vi "init_chessboard.vi"(8 "error in (no error)":errorcluster, 10 "starting_square":T1, 11 "chessboard_size":u8) -> (0 "error out":errorcluster, 3 "chessboard (populated)":T2[][](array[typedef]))   [LabVIEW 2020, in "core.lvlib"]
uses:
  core.lvlib
  core_data/core_data.ctl
  core_data/tour_in_progress.ctl
  core_data/chessboard_index.ctl
  core_data/chess_square.ctl
  core_data/neighbour_square.ctl
  core_data/core_data.lvlib
  PTRL/errors/errors.lvlib
panel:
  out "no. of neighbours":i32[][](array[numeric])
  out "no. of rows and columns":i32[](array[numeric])
  out "chessboard (not populated)":T2[][](array[typedef])
  out "chess_square":T2
  out "core_data":T4
  # "Development\ncontrols/indicators useful for development and testing, but which are not outputs of the VI"
  # "Input\nInputs to the VI"
  # "Output\nOutputs of the VI"
  # "Description\n\nBlank VI with error handling case. \n\nSummarize the use of this VI in this space."
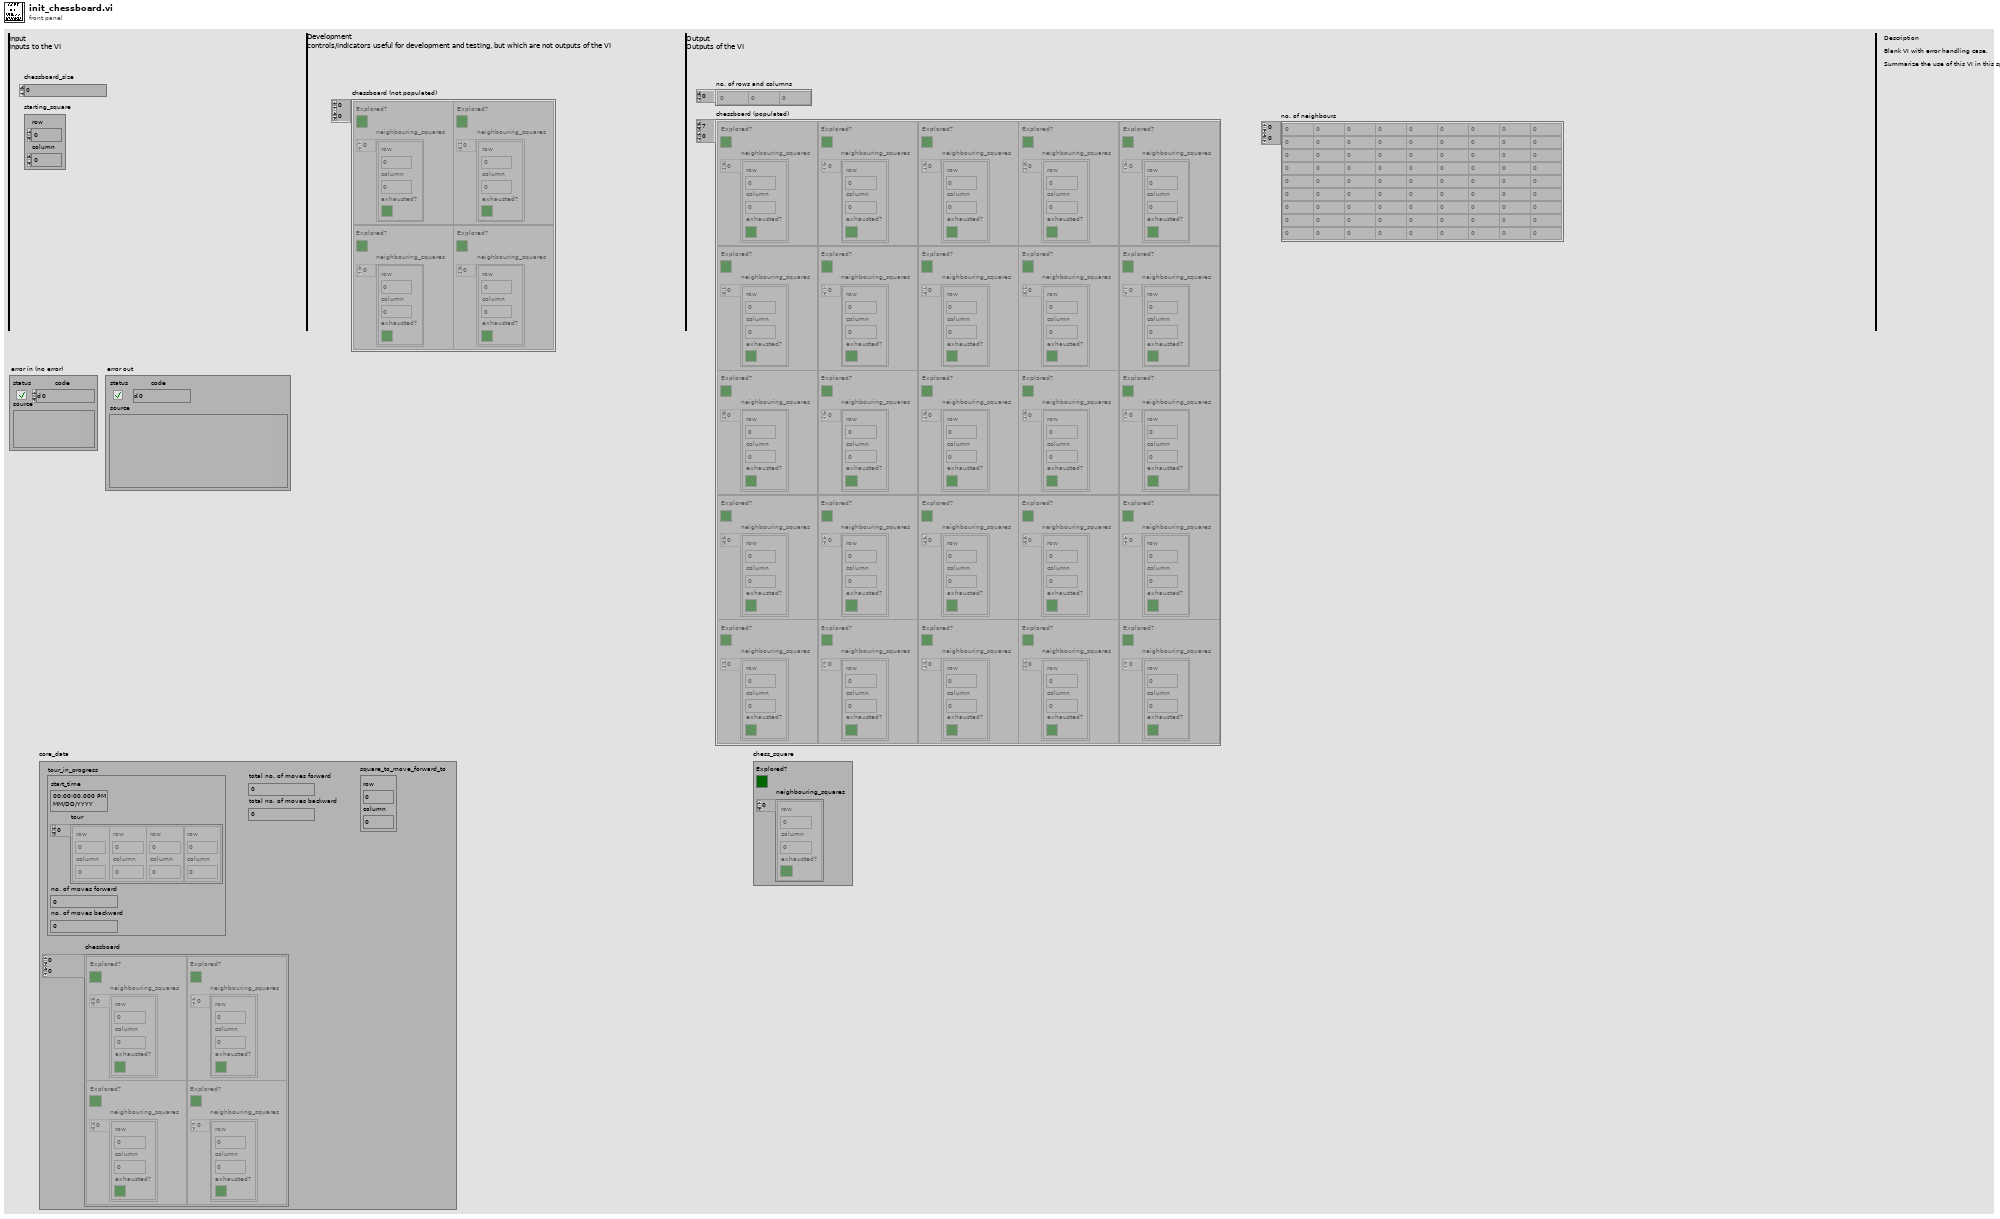
[diagram p1: front panel]
types:
  T1 = typedef "core.lvlib/core_data.lvlib/chessboard_index.ctl" = cluster{"row":u8, "column":u8}
  T2 = typedef "core.lvlib/core_data.lvlib/chess_square.ctl" = cluster{"Explored?":bool, "neighbouring_squares":T3[]}
  T3 = typedef "core.lvlib/core_data.lvlib/neighbour_square.ctl" = cluster{"row":u8, "column":u8, "exhausted?":bool}
  T4 = typedef "core.lvlib/core_data.lvlib/core_data.ctl" = cluster{"tour_in_progress":T5, "total no. of moves forward":u64, "total no. of moves backward":u64, "chessboard":T2[][], "square_to_move_forward_to":T1}
  T5 = typedef "core.lvlib/core_data.lvlib/tour_in_progress.ctl" = cluster{"start_time":timestamp, "tour":T1[], "no. of moves forward":u64, "no. of moves backward":u64}
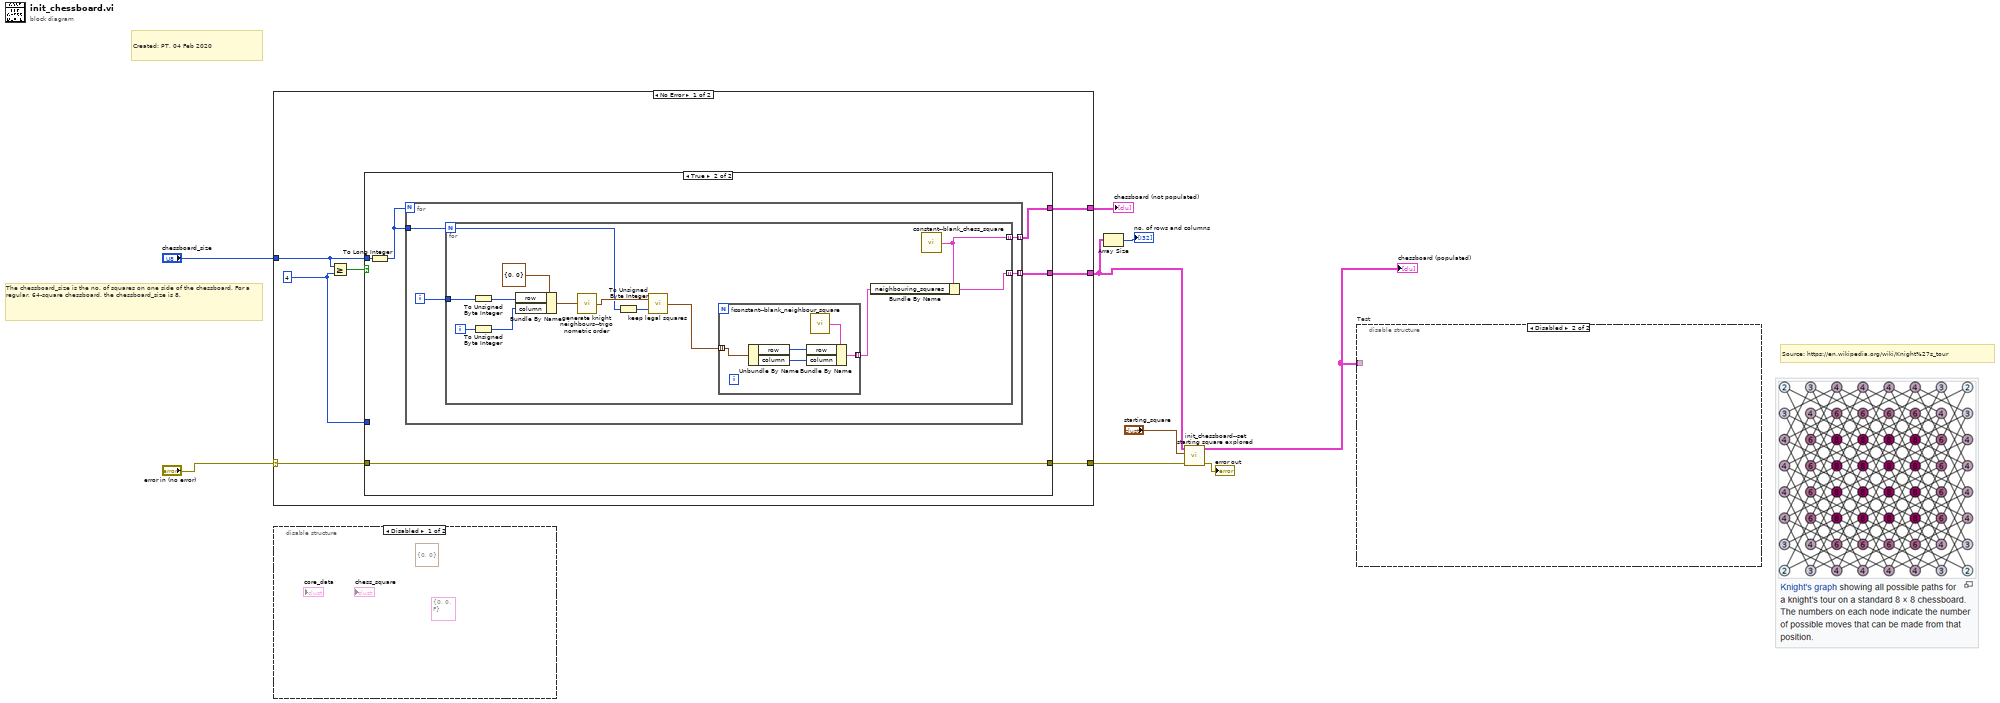
[diagram p0: block diagram]
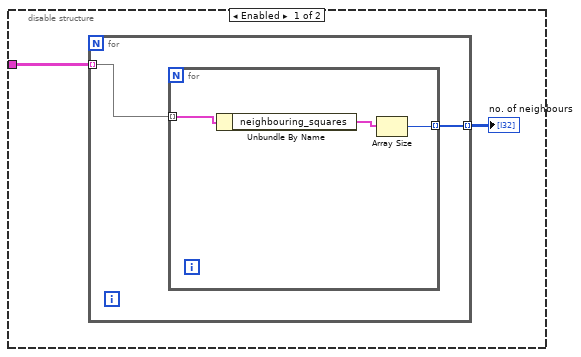
[diagram p2: hidden frame]
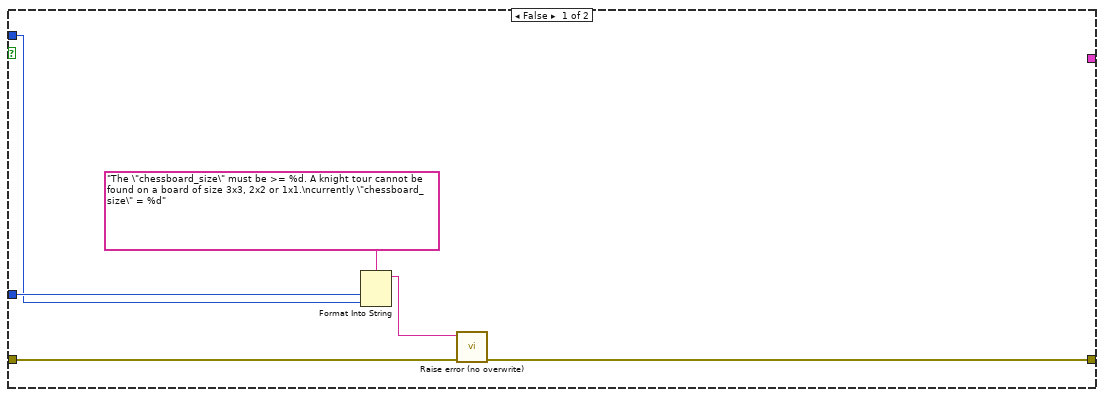
[diagram p4: hidden frame]
diagram:
  # "Source: https://en.wikipedia.org/wiki/Knight%27s_tour"
  # "The chessboard_size is the no. of squares on one side of the chessboard. For a regular, 64-square chessboard, the chessboard_size is 8."
  # "Created: PT, 04 Feb 2020"
  n1 = case shown="No Error" "error in (no error)" {
    selector: "error in (no error)" -> [w14 w50]
    tunnel: [w13 w50] -> w3
    tunnel: "chessboard_size" -> [w16 _]
    tunnel: [w11 _] -> w7
    tunnel: [w10 _] -> w5
    frame No Error {
      w12 = u8 4 ("y")
      n2 = Greater Or Equal?(x=w16, y=w12) -> (x >= y?=w15:bool)
      n3 = case shown="True" w15 {
        tunnel: w16 -> [w17 w27]
        tunnel: w14 -> [w22 w25]
        tunnel: [w21 w25] -> w13
        tunnel: w12 -> [w18 _]
        tunnel: [_ w24] -> w11
        tunnel: [_ w23] -> w10
        frame False {
          n4 = Format Into String(format string="The \"chessboard_size\" must be >= %d. A knight tour cannot be found on a board of size 3x3, 2x2 or 1x1.\ncurrently \"chessboard_size\" = %d", w18, w17) -> (resulting string=w19:string)  [unwired: 2 in, 1 out]
          n5 = call "Raise error (no overwrite).vi"("error in"=w22, "error message (\"\")"=w19) -> ("error out"=w21:errorcluster)  [unwired: 9 in]
        }
        frame True {
          n6 = To Long Integer(number=w27) -> (32bit integer=w26:i32)
          n7 = for {
            N: w26 -> [_]
            tunnel: w26 -> [w31]
            tunnel: [w30] -> w23 mode=indexing
            tunnel: [w28] -> w24 mode=indexing
            i -> [w29]
            n8 = for {
              N: w31 -> [w37]
              tunnel: [w32] -> w30 mode=indexing
              tunnel: w29 -> [w43]
              tunnel: [w33] -> w28 mode=indexing
              i -> [w42]
              n9 = To Unsigned Byte Integer(number=w43) -> (unsigned 8bit integer=w41:u8)
              n10 = To Unsigned Byte Integer(number=w42) -> (unsigned 8bit integer=w40:u8)
              n11 = Bundle By Name(cluster=T1 {"row"=0, "column"=0} ("chessboard_index"), "row"=w41, "column"=w40) -> (w39:T1)
              n12 = call "generate knight neighbours--trigonometric order.vi"("current square (chessboard_index)"=w39) -> ("neighbours (chessboard_index)"=w38:T1[])
              n13 = To Unsigned Byte Integer(number=w37) -> (unsigned 8bit integer=w36:u8)
              n14 = call "keep legal squares.vi"("chessboard_size"=w36, "squares (chessboard_index)"=w38) -> ("legal squares only (chessboard_index)"=w35:T1[])
              n15 = for {
                tunnel: w35 -> [w48] mode=indexing
                tunnel: [w45] -> w34 mode=indexing
                n16 = Unbundle By Name(w48) -> ("row"=w47:u8, "column"=w46:u8)
                n17 = call "constant--blank_neighbour_square.vi"() -> ("blank_neighbour_square"=w49:T3)
                n18 = Bundle By Name(cluster=w49, "row"=w47, "column"=w46) -> (w45:T3)
              }
              n19 = call "constant--blank_chess_square.vi"() -> ("blank_chess_square"=w33:T2)
              n20 = Bundle By Name(cluster=w33, "neighbouring_squares"=w34) -> (w32:T2)
            }
          }
        }
      }
    }
    frame Error {
    }
  }
  "chessboard (not populated)" <- w7
  n21 = disable-structure shown="Disabled" {
    frame Disabled {
      (unwired) T3 {"row"=0, "column"=0, "exhausted?"=FALSE} ("neighbour_square")
      (unwired) T1 {"row"=0, "column"=0} ("chessboard_index")
    }
    frame Enabled {
    }
  }
  n22 = Array Size(array=w5) -> (size(s)=→"no. of rows and columns":i32[])
  n23 = call "init_chessboard--set starting square explored.vi"("error in (no error)"=w3, "starting_square"="starting_square", "chessboard in"=w5) -> ("error out"=→"error out":errorcluster, "chessboard out (starting square marked as explored)"=w1:T2[][])  [unwired: 7 in]
  "chessboard (populated)" <- w1
  n24 = disable-structure "Test" shown="Disabled" {
    disable-tunnel: w1 -> [w52 _]
    frame Enabled {
      n25 = for {
        tunnel: w52 -> [w54] mode=indexing
        tunnel: [w53] -> w51 mode=indexing
        n26 = for {
          tunnel: w54 -> [w57] mode=indexing
          tunnel: [w55] -> w53 mode=indexing
          n27 = Unbundle By Name(w57) -> ("neighbouring_squares"=w56:T3[])
          n28 = Array Size(array=w56) -> (size(s)=w55:i32)
        }
      }
      "no. of neighbours" <- w51
    }
    frame Disabled {
    }
  }
